vi "DAQ_Route synchronization signals.vi"(0 "DAQmx Task In":refnum<k21>, 5 "Routing paths":T1[](array[typedef]), 11 "error in":errorcluster) -> (4 "DAQmx Task Out":refnum<k21>, 15 "error out":errorcluster)   [LabVIEW 2021, in "DAQ_Synchronization.lvlib"]
doc: "<B>Route synchronization signals</B> VI can be used to route signal between specified signal and output terminal. \n\nThe specified source signal and output terminal can be on different devices as long as a connecting public bus, such as TestScale backplane, connects the devices. These routes are embedded in a task. When the task is committed, the route is committed. When the task is cleared, the route is unreserved."
uses:
  DAQ_Synchronization.lvlib
  Typedefs/Routing Path.ctl
  Typedefs/Routing Signal.ctl
  <vilib>/DAQmx/configure/events/hardwareSignals.llb/DAQmx Export Signal (Most Signals).vi
panel:
  # "Inputs"
  # "Outputs"
  # "Overview:\nThis VI determines device routing of various paths between specified exported signal and output terminal. These routes are embedded in the DAQmx task.\n\nHardware Requirements: A compatible PXI, PCIe, USB, cDAQ or Testscale device\n\nSoftware Requirements: NI DAQmx 2022 Q4 or later\n\nInstructions:\n1. Input the task reference in DAQmx Task In control to perfrom routing.\n2. Enter Routing paths between source signal and output terminal to perform connection. Refer to the Device Routes table in Measurement and Automation Explorer to determine eligible signals and terminals for routing. \n\nNote: \n1. The source signal and output terminals can be on different devices as long as a connecting public bus, such as TestScale backplane, connects the devices. \n2. The routes created by this VI are embedded in a task. This routing is termed as Task-Based Routing. When the task is committed, the route is committed. When the task is cleared, the route is unreserved."
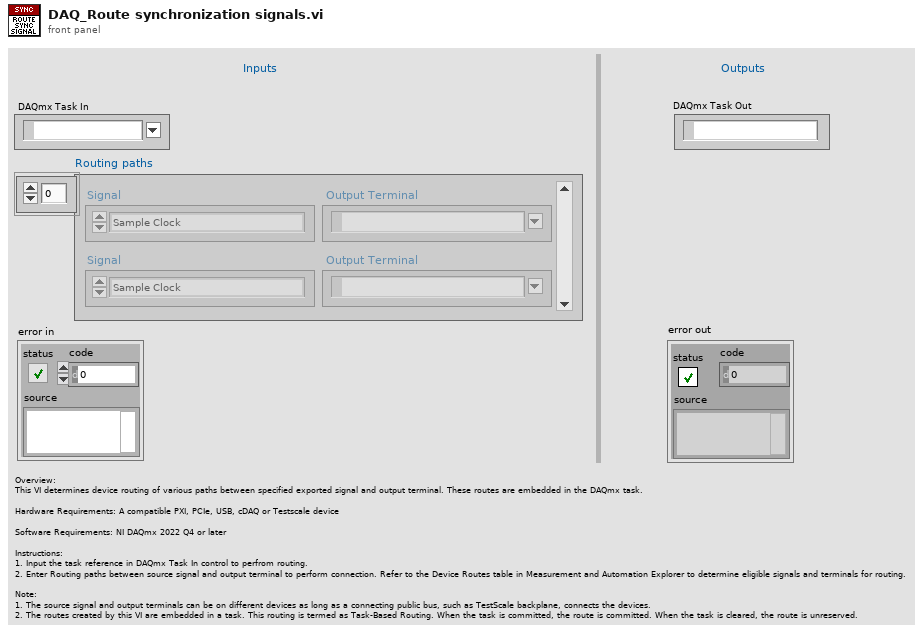
[diagram p1: front panel]
types:
  T1 = typedef "DAQ_Synchronization.lvlib/Routing Path.ctl" = cluster{"Signal":T2, "Output Terminal":tag}
  T2 = typedef "DAQ_Synchronization.lvlib/Routing Signal.ctl" = enum16{"Sample Clock", "Start Trigger"}
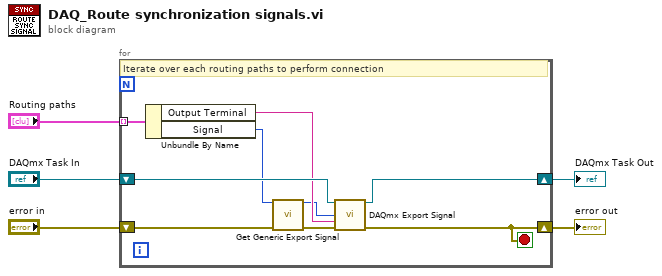
[diagram p0: block diagram]
diagram:
  n1 = for {
    shift-right: [w7] -> w4
    shift-left: "error in" -> [w10]
    tunnel: "Routing paths" -> [w12] mode=indexing
    shift-right: [w14] -> w1
    shift-left: "DAQmx Task In" -> [w13]
    stop <- w7 stop-if-true
    # "Iterate over each routing paths to perform connection"
    n2 = Unbundle By Name(w12) -> ("Output Terminal"=w8:tag, "Signal"=w11:T2)
    n3 = call "Get Generic Export Signal.vi"("Signal In"=w11, "error in"=w10) -> ("Generic Signal Out"=w6:i32, "error out"=w9:errorcluster)  [unwired: 12 in]
    n4 = call-poly <vilib>:"DAQmx Export Signal.vi"("task/channels in"=w13, "signal"=w6, "output terminal"=w8, "error in"=w9) -> ("task out"=w14:refnum<k21>, "error out"=w7:errorcluster)  [unwired: 10 in]
  }
  "error out" <- w4
  "DAQmx Task Out" <- w1
